vi "updateErrorCode.vi"(8 "error in (no error)":errorcluster, 11 "Model in":refnum<class "Model.lvclass">) -> (0 "error out":errorcluster, 3 "Model out":refnum<class "Model.lvclass">)   [LabVIEW 2013, in "Model.lvclass"]
uses:
  Model.lvclass
  Model.lvclass/Model.ctl
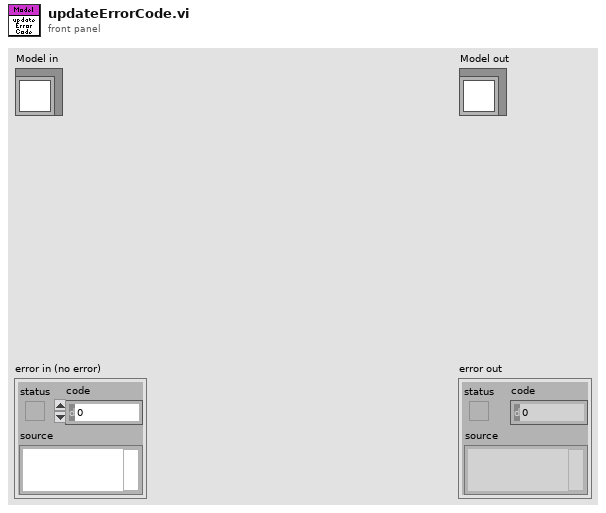
[diagram p1: front panel]
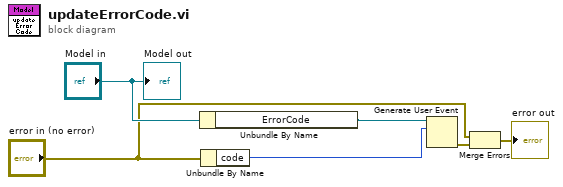
[diagram p0: block diagram]
diagram:
  n1 = Unbundle By Name("Model in") -> ("ErrorCode"=w5:refnum<user-event>)
  n2 = Unbundle By Name("error in (no error)") -> ("code"=w4:i32)
  n3 = Generate User Event(user event=w5, event data cluster=w4) -> (error out=w2:errorcluster)  [unwired: 2 in, 1 out]
  n4 = Merge Errors("error in (no error)", w2) -> (→"error out":errorcluster)
  "Model out" <- "Model in"
